vi "大富翁.vi"() -> ()   [LabVIEW 2014] (continued)
                                n1877 = stacked-sequence {
                                tunnel: [_ w1316] -> w1303
                                frame #0 {
                                n1878 = call "機會-500.vi"() -> ()  [unwired: 4 in]
                                n1879 = local read "換誰?"() -> (w1304:dbl)
                                n1880 = case shown="1, Default" w1304 {
                                tunnel: [w1312 w1313 w1314 w1315] -> w1305
                                frame 1, Default {
                                n1881 = local read "玩家一財產"() -> (w1312:dbl)
                                }
                                frame 2 {
                                n1882 = local read "玩家二財產"() -> (w1313:dbl)
                                }
                                frame 3 {
                                n1883 = local read "玩家三財產"() -> (w1314:dbl)
                                }
                                frame 4 {
                                n1884 = local read "玩家四財產"() -> (w1315:dbl)
                                }
                                }
                                n1885 = Subtract(x=w1305, y=500.0) -> (x-y=w1307:dbl)
                                n1886 = case shown="1, Default" w1304 {
                                tunnel: w1307 -> [w1308 w1309 w1310 w1311]
                                frame 1, Default {
                                n1887 = local write "玩家一財產"(w1308) -> ()
                                }
                                frame 2 {
                                n1888 = local write "玩家二財產"(w1309) -> ()
                                }
                                frame 3 {
                                n1889 = local write "玩家三財產"(w1310) -> ()
                                }
                                frame 4 {
                                n1890 = local write "玩家四財產"(w1311) -> ()
                                }
                                }
                                }
                                frame #1 {
                                n1891 = local read "換誰?"() -> (w1318:dbl)
                                n1892 = case shown="1, Default" w1318 {
                                tunnel: [w1322 w1323 w1324 w1325] -> w1319
                                frame 1, Default {
                                n1893 = local read "玩家一財產"() -> (w1322:dbl)
                                }
                                frame 2 {
                                n1894 = local read "玩家二財產"() -> (w1323:dbl)
                                }
                                frame 3 {
                                n1895 = local read "玩家三財產"() -> (w1324:dbl)
                                }
                                frame 4 {
                                n1896 = local read "玩家四財產"() -> (w1325:dbl)
                                }
                                }
                                n1897 = Less Than 0?(x=w1319) -> (x < 0?=w1317:bool)
                                n1898 = case shown="True" w1317 {
                                tunnel: [FALSE TRUE] -> w1316
                                frame False {
                                }
                                frame True {
                                n1899 = call "破產了.vi"() -> ()  [unwired: 4 in]
                                }
                                }
                                }
                                }
                                }
                                }
                                }
                                frame True {
                                # "58~60"
                                n1900 = call "機會全部+3000.vi"() -> ()  [unwired: 4 in]
                                n1901 = local read "玩家三財產"() -> (w1330:dbl)
                                n1902 = local read "玩家二財產"() -> (w1332:dbl)
                                n1903 = local read "玩家一財產"() -> (w1334:dbl)
                                n1904 = Add(x=w1330, y=3000.0) -> (x+y=w1329:dbl)
                                n1905 = Add(x=w1332, y=3000.0) -> (x+y=w1331:dbl)
                                n1906 = local read "玩家四財產"() -> (w1328:dbl)
                                n1907 = Add(x=w1334, y=3000.0) -> (x+y=w1333:dbl)
                                n1908 = Add(x=w1328, y=3000.0) -> (x+y=w1327:dbl)
                                n1909 = local write "玩家三財產"(w1329) -> ()
                                n1910 = local write "玩家二財產"(w1331) -> ()
                                n1911 = local write "玩家四財產"(w1327) -> ()
                                n1912 = local write "玩家一財產"(w1333) -> ()
                                }
                                }
                                }
                                frame True {
                                # "54~58"
                                n1913 = call "機會+3000.vi"() -> ()  [unwired: 4 in]
                                n1914 = local read "換誰?"() -> (w1340:dbl)
                                n1915 = case shown="1, Default" w1340 {
                                tunnel: [w1348 w1349 w1350 w1351] -> w1341
                                frame 1, Default {
                                n1916 = local read "玩家一財產"() -> (w1348:dbl)
                                }
                                frame 2 {
                                n1917 = local read "玩家二財產"() -> (w1349:dbl)
                                }
                                frame 3 {
                                n1918 = local read "玩家三財產"() -> (w1350:dbl)
                                }
                                frame 4 {
                                n1919 = local read "玩家四財產"() -> (w1351:dbl)
                                }
                                }
                                n1920 = Add(x=w1341, y=3000.0) -> (x+y=w1343:dbl)
                                n1921 = case shown="1, Default" w1340 {
                                tunnel: w1343 -> [w1344 w1345 w1346 w1347]
                                frame 1, Default {
                                n1922 = local write "玩家一財產"(w1344) -> ()
                                }
                                frame 2 {
                                n1923 = local write "玩家二財產"(w1345) -> ()
                                }
                                frame 3 {
                                n1924 = local write "玩家三財產"(w1346) -> ()
                                }
                                frame 4 {
                                n1925 = local write "玩家四財產"(w1347) -> ()
                                }
                                }
                                }
                                }
                                }
                                frame True {
                                # "45~54"
                                n1926 = call "機會+2000.vi"() -> ()  [unwired: 4 in]
                                n1927 = local read "換誰?"() -> (w1353:dbl)
                                n1928 = case shown="1, Default" w1353 {
                                tunnel: [w1361 w1362 w1363 w1364] -> w1354
                                frame 1, Default {
                                n1929 = local read "玩家一財產"() -> (w1361:dbl)
                                }
                                frame 2 {
                                n1930 = local read "玩家二財產"() -> (w1362:dbl)
                                }
                                frame 3 {
                                n1931 = local read "玩家三財產"() -> (w1363:dbl)
                                }
                                frame 4 {
                                n1932 = local read "玩家四財產"() -> (w1364:dbl)
                                }
                                }
                                n1933 = Add(x=w1354, y=2000.0) -> (x+y=w1356:dbl)
                                n1934 = case shown="1, Default" w1353 {
                                tunnel: w1356 -> [w1357 w1358 w1359 w1360]
                                frame 1, Default {
                                n1935 = local write "玩家一財產"(w1357) -> ()
                                }
                                frame 2 {
                                n1936 = local write "玩家二財產"(w1358) -> ()
                                }
                                frame 3 {
                                n1937 = local write "玩家三財產"(w1359) -> ()
                                }
                                frame 4 {
                                n1938 = local write "玩家四財產"(w1360) -> ()
                                }
                                }
                                }
                                }
                                }
                                frame True {
                                # "30~45"
                                n1939 = call "機會+1000.vi"() -> ()  [unwired: 4 in]
                                n1940 = local read "換誰?"() -> (w1366:dbl)
                                n1941 = case shown="1, Default" w1366 {
                                tunnel: [w1374 w1375 w1376 w1377] -> w1367
                                frame 1, Default {
                                n1942 = local read "玩家一財產"() -> (w1374:dbl)
                                }
                                frame 2 {
                                n1943 = local read "玩家二財產"() -> (w1375:dbl)
                                }
                                frame 3 {
                                n1944 = local read "玩家三財產"() -> (w1376:dbl)
                                }
                                frame 4 {
                                n1945 = local read "玩家四財產"() -> (w1377:dbl)
                                }
                                }
                                n1946 = Add(x=w1367, y=1000.0) -> (x+y=w1369:dbl)
                                n1947 = case shown="1, Default" w1366 {
                                tunnel: w1369 -> [w1370 w1371 w1372 w1373]
                                frame 1, Default {
                                n1948 = local write "玩家一財產"(w1370) -> ()
                                }
                                frame 2 {
                                n1949 = local write "玩家二財產"(w1371) -> ()
                                }
                                frame 3 {
                                n1950 = local write "玩家三財產"(w1372) -> ()
                                }
                                frame 4 {
                                n1951 = local write "玩家四財產"(w1373) -> ()
                                }
                                }
                                }
                                }
                              }
                              frame True {
                                # "10~30"
                                n1952 = call "機會+500.vi"() -> ()  [unwired: 4 in]
                                n1953 = local read "換誰?"() -> (w1382:dbl)
                                n1954 = case shown="1, Default" w1382 {
                                tunnel: [w1387 w1388 w1389 w1390] -> w1381
                                frame 1, Default {
                                n1955 = local read "玩家一財產"() -> (w1387:dbl)
                                }
                                frame 2 {
                                n1956 = local read "玩家二財產"() -> (w1388:dbl)
                                }
                                frame 3 {
                                n1957 = local read "玩家三財產"() -> (w1389:dbl)
                                }
                                frame 4 {
                                n1958 = local read "玩家四財產"() -> (w1390:dbl)
                                }
                                }
                                n1959 = Add(x=w1381, y=500.0) -> (x+y=w1379:dbl)
                                n1960 = case shown="4" w1382 {
                                tunnel: w1379 -> [w1383 w1384 w1385 w1386]
                                frame 1, Default {
                                n1961 = local write "玩家一財產"(w1383) -> ()
                                }
                                frame 2 {
                                n1962 = local write "玩家二財產"(w1384) -> ()
                                }
                                frame 3 {
                                n1963 = local write "玩家三財產"(w1385) -> ()
                                }
                                frame 4 {
                                n1964 = local write "玩家四財產"(w1386) -> ()
                                }
                                }
                              }
                            }
                          }
                          frame True {
                            # "5~10%"
                            n1965 = local read "換誰?"() -> (w1392:dbl)
                            n1966 = case shown="1" w1392 {
                              frame 0, Default {
                              }
                              frame 1 {
                                n1967 = local write "剩幾天 1"(2.0 ("剩幾天 1")) -> ()
                                n1968 = local write "位置 1"(13.0 ("位置 1")) -> ()
                                n1969 = property on="入獄 1" class="Bool (strict)"("Visible"=TRUE) -> ()  [unwired: 2 in, 2 out]
                                n1970 = property on="P1 棋子" class="Bool (strict)"("Left"=1503 ("Position:Left"), "Top"=112 ("Position:Top")) -> ()  [unwired: 2 in, 2 out]
                              }
                              frame 2 {
                                n1971 = local write "位置 2"(13.0 ("位置 2")) -> ()
                                n1972 = local write "剩幾天 2"(2.0 ("剩幾天 2")) -> ()
                                n1973 = property on="入獄 2" class="Bool (strict)"("Visible"=TRUE) -> ()  [unwired: 2 in, 2 out]
                                n1974 = property on="P2 棋子" class="Bool (strict)"("Left"=1540 ("Position:Left"), "Top"=112 ("Position:Top")) -> ()  [unwired: 2 in, 2 out]
                              }
                              frame 3 {
                                n1975 = local write "剩幾天 3"(2.0 ("剩幾天 3")) -> ()
                                n1976 = local write "位置 3"(13.0 ("位置 3")) -> ()
                                n1977 = property on="入獄 3" class="Bool (strict)"("Visible"=TRUE) -> ()  [unwired: 2 in, 2 out]
                                n1978 = property on="P3 棋子" class="Bool (strict)"("Left"=1503 ("Position:Left"), "Top"=144 ("Position:Top")) -> ()  [unwired: 2 in, 2 out]
                              }
                              frame 4 {
                                n1979 = local write "剩幾天 4"(2.0 ("剩幾天 4")) -> ()
                                n1980 = local write "位置 4"(13.0 ("位置 4")) -> ()
                                n1981 = property on="入獄 4" class="Bool (strict)"("Visible"=TRUE) -> ()  [unwired: 2 in, 2 out]
                                n1982 = property on="P4 棋子" class="Bool (strict)"("Left"=1540 ("Position:Left"), "Top"=144 ("Position:Top")) -> ()  [unwired: 2 in, 2 out]
                              }
                            }
                            n1983 = call "32入獄.vi"() -> ()  [unwired: 4 in]
                          }
                        }
                      }
                      frame True {
                        # "2~5"
                        n1984 = local read "換誰?"() -> (w1414:dbl)
                        n1985 = case shown="1" w1414 {
                          frame 0, Default {
                          }
                          frame 1 {
                            n1986 = local write "剩幾天 1"(3.0 ("剩幾天 1")) -> ()
                            n1987 = local write "位置 1"(13.0 ("位置 1")) -> ()
                            n1988 = property on="入獄 1" class="Bool (strict)"("Visible"=TRUE) -> ()  [unwired: 2 in, 2 out]
                            n1989 = property on="P1 棋子" class="Bool (strict)"("Left"=1503 ("Position:Left"), "Top"=112 ("Position:Top")) -> ()  [unwired: 2 in, 2 out]
                          }
                          frame 2 {
                            n1990 = local write "位置 2"(13.0 ("位置 2")) -> ()
                            n1991 = local write "剩幾天 2"(3.0 ("剩幾天 2")) -> ()
                            n1992 = property on="入獄 2" class="Bool (strict)"("Visible"=TRUE) -> ()  [unwired: 2 in, 2 out]
                            n1993 = property on="P2 棋子" class="Bool (strict)"("Left"=1540 ("Position:Left"), "Top"=112 ("Position:Top")) -> ()  [unwired: 2 in, 2 out]
                          }
                          frame 3 {
                            n1994 = local write "剩幾天 3"(3.0 ("剩幾天 3")) -> ()
                            n1995 = local write "位置 3"(13.0 ("位置 3")) -> ()
                            n1996 = property on="入獄 3" class="Bool (strict)"("Visible"=TRUE) -> ()  [unwired: 2 in, 2 out]
                            n1997 = property on="P3 棋子" class="Bool (strict)"("Left"=1503 ("Position:Left"), "Top"=144 ("Position:Top")) -> ()  [unwired: 2 in, 2 out]
                          }
                          frame 4 {
                            n1998 = local write "剩幾天 4"(3.0 ("剩幾天 4")) -> ()
                            n1999 = local write "位置 4"(13.0 ("位置 4")) -> ()
                            n2000 = property on="入獄 4" class="Bool (strict)"("Visible"=TRUE) -> ()  [unwired: 2 in, 2 out]
                            n2001 = property on="P4 棋子" class="Bool (strict)"("Left"=1540 ("Position:Left"), "Top"=144 ("Position:Top")) -> ()  [unwired: 2 in, 2 out]
                          }
                        }
                        n2002 = call "入獄3天.vi"() -> ()  [unwired: 4 in]
                      }
                    }
                  }
                  frame True {
                    # "0~2%"
                    n2003 = stacked-sequence {
                      tunnel: [_ w1468] -> w1435
                      frame #0 {
                        n2004 = local read "換誰?"() -> (w1436:dbl)
                        n2005 = case shown="4" w1436 {
                          frame 0, Default {
                          }
                          frame 1 {
                            n2006 = local write "剩幾天 1"(5.0 ("剩幾天 1")) -> ()
                            n2007 = local write "位置 1"(13.0 ("位置 1")) -> ()
                            n2008 = property on="入獄 1" class="Bool (strict)"("Visible"=TRUE) -> ()  [unwired: 2 in, 2 out]
                            n2009 = property on="P1 棋子" class="Bool (strict)"("Left"=1503 ("Position:Left"), "Top"=112 ("Position:Top")) -> ()  [unwired: 2 in, 2 out]
                          }
                          frame 2 {
                            n2010 = local write "位置 2"(13.0 ("位置 2")) -> ()
                            n2011 = local write "剩幾天 2"(5.0 ("剩幾天 2")) -> ()
                            n2012 = property on="入獄 2" class="Bool (strict)"("Visible"=TRUE) -> ()  [unwired: 2 in, 2 out]
                            n2013 = property on="P2 棋子" class="Bool (strict)"("Left"=1540 ("Position:Left"), "Top"=112 ("Position:Top")) -> ()  [unwired: 2 in, 2 out]
                          }
                          frame 3 {
                            n2014 = local write "剩幾天 3"(5.0 ("剩幾天 3")) -> ()
                            n2015 = local write "位置 3"(13.0 ("位置 3")) -> ()
                            n2016 = property on="入獄 3" class="Bool (strict)"("Visible"=TRUE) -> ()  [unwired: 2 in, 2 out]
                            n2017 = property on="P3 棋子" class="Bool (strict)"("Left"=1503 ("Position:Left"), "Top"=144 ("Position:Top")) -> ()  [unwired: 2 in, 2 out]
                          }
                          frame 4 {
                            n2018 = local write "剩幾天 4"(5.0 ("剩幾天 4")) -> ()
                            n2019 = local write "位置 4"(13.0 ("位置 4")) -> ()
                            n2020 = property on="入獄 4" class="Bool (strict)"("Visible"=TRUE) -> ()  [unwired: 2 in, 2 out]
                            n2021 = property on="P4 棋子" class="Bool (strict)"("Left"=1540 ("Position:Left"), "Top"=144 ("Position:Top")) -> ()  [unwired: 2 in, 2 out]
                          }
                        }
                        n2022 = case shown="1, Default" w1436 {
                          tunnel: [w1444 w1445 w1446 w1447] -> w1439
                          frame 1, Default {
                            n2023 = local read "玩家一財產"() -> (w1444:dbl)
                          }
                          frame 2 {
                            n2024 = local read "玩家二財產"() -> (w1445:dbl)
                          }
                          frame 3 {
                            n2025 = local read "玩家三財產"() -> (w1446:dbl)
                          }
                          frame 4 {
                            n2026 = local read "玩家四財產"() -> (w1447:dbl)
                          }
                        }
                        n2027 = Subtract(x=w1439, y=2000.0) -> (x-y=w1437:dbl)
                        n2028 = case shown="4" w1436 {
                          tunnel: w1437 -> [w1440 w1441 w1442 w1443]
                          frame 1, Default {
                            n2029 = local write "玩家一財產"(w1440) -> ()
                          }
                          frame 2 {
                            n2030 = local write "玩家二財產"(w1441) -> ()
                          }
                          frame 3 {
                            n2031 = local write "玩家三財產"(w1442) -> ()
                          }
                          frame 4 {
                            n2032 = local write "玩家四財產"(w1443) -> ()
                          }
                        }
                        n2033 = call "入獄5天.vi"() -> ()  [unwired: 4 in]
                      }
                      frame #1 {
                        n2034 = local read "換誰?"() -> (w1470:dbl)
                        n2035 = case shown="1, Default" w1470 {
                          tunnel: [w1474 w1475 w1476 w1477] -> w1471
                          frame 1, Default {
                            n2036 = local read "玩家一財產"() -> (w1474:dbl)
                          }
                          frame 2 {
                            n2037 = local read "玩家二財產"() -> (w1475:dbl)
                          }
                          frame 3 {
                            n2038 = local read "玩家三財產"() -> (w1476:dbl)
                          }
                          frame 4 {
                            n2039 = local read "玩家四財產"() -> (w1477:dbl)
                          }
                        }
                        n2040 = Less Than 0?(x=w1471) -> (x < 0?=w1469:bool)
                        n2041 = case shown="True" w1469 {
                          tunnel: [FALSE TRUE] -> w1468
                          frame False {
                          }
                          frame True {
                            n2042 = call "破產了.vi"() -> ()  [unwired: 4 in]
                          }
                        }
                      }
                    }
                  }
                }
              }
              frame True {
                n2043 = local read "換誰?"() -> (w1479:dbl)
                n2044 = case shown="4" w1479 {
                  frame 0, Default {
                  }
                  frame 1 {
                    n2045 = local write "剩幾天 1"(2.0 ("剩幾天 1")) -> ()
                    n2046 = local write "位置 1"(13.0 ("位置 1")) -> ()
                    n2047 = property on="入獄 1" class="Bool (strict)"("Visible"=TRUE) -> ()  [unwired: 2 in, 2 out]
                    n2048 = property on="P1 棋子" class="Bool (strict)"("Left"=1503 ("Position:Left"), "Top"=112 ("Position:Top")) -> ()  [unwired: 2 in, 2 out]
                  }
                  frame 2 {
                    n2049 = local write "剩幾天 2"(2.0 ("剩幾天 2")) -> ()
                    n2050 = local write "位置 2"(13.0 ("位置 2")) -> ()
                    n2051 = property on="入獄 2" class="Bool (strict)"("Visible"=TRUE) -> ()  [unwired: 2 in, 2 out]
                    n2052 = property on="P2 棋子" class="Bool (strict)"("Left"=1540 ("Position:Left"), "Top"=112 ("Position:Top")) -> ()  [unwired: 2 in, 2 out]
                  }
                  frame 3 {
                    n2053 = local write "剩幾天 3"(2.0 ("剩幾天 3")) -> ()
                    n2054 = local write "位置 3"(13.0 ("位置 3")) -> ()
                    n2055 = local write "位置 3"(13.0 ("位置 3")) -> ()
                    n2056 = property on="入獄 3" class="Bool (strict)"("Visible"=TRUE) -> ()  [unwired: 2 in, 2 out]
                    n2057 = property on="P3 棋子" class="Bool (strict)"("Left"=1503 ("Position:Left"), "Top"=144 ("Position:Top")) -> ()  [unwired: 2 in, 2 out]
                  }
                  frame 4 {
                    n2058 = local write "位置 4"(13.0 ("位置 4")) -> ()
                    n2059 = local write "剩幾天 4"(2.0 ("剩幾天 4")) -> ()
                    n2060 = property on="入獄 4" class="Bool (strict)"("Visible"=TRUE) -> ()  [unwired: 2 in, 2 out]
                    n2061 = property on="P4 棋子" class="Bool (strict)"("Left"=1540 ("Position:Left"), "Top"=144 ("Position:Top")) -> ()  [unwired: 2 in, 2 out]
                  }
                }
                n2062 = call "32入獄.vi"() -> ()  [unwired: 4 in]
              }
            }
          }
          frame 9 {
            n2063 = local read "台東縣所有"() -> (w1501:u32)
            n2064 = Equal?(x=w1501, y=u32 16777215) -> (x = y?=w1504:bool)
            n2065 = case shown="False" w1504 {
              tunnel: w1503 -> [w1528 w1565]
              tunnel: [w1518 FALSE] -> w1502
              frame False {
                # "有主地"
                n2066 = local read "換誰?"() -> (w1521:dbl)
                n2067 = local read "台東縣所有"() -> (w1507:u32)
                n2068 = call "數字轉顏色.vi"("數字"=w1521) -> ("顏色數字"=w1508:dbl)  [unwired: 2 in]
                n2069 = case shown="4" w1521 {
                  tunnel: [w1560 w1561 w1562 w1563] -> w1527
                  frame 1, Default {
                    n2070 = local read "玩家一財產"() -> (w1560:dbl)
                  }
                  frame 2 {
                    n2071 = local read "玩家二財產"() -> (w1561:dbl)
                  }
                  frame 3 {
                    n2072 = local read "玩家三財產"() -> (w1562:dbl)
                  }
                  frame 4 {
                    n2073 = local read "玩家四財產"() -> (w1563:dbl)
                  }
                }
                n2074 = Equal?(x=w1507, y=w1508) -> (x = y?=w1531:bool)
                n2075 = local read "台東縣所有"() -> (w1509:u32)
                n2076 = local read "9旅4"() -> (w1517:bool)
                n2077 = local read "9旅3"() -> (w1516:bool)
                n2078 = local read "9旅2"() -> (w1515:bool)
                n2079 = local read "9旅1"() -> (w1514:bool)
                n2080 = local read "9房4"() -> (w1513:bool)
                n2081 = local read "9房3"() -> (w1512:bool)
                n2082 = local read "9房2"() -> (w1511:bool)
                n2083 = local read "9房1"() -> (w1510:bool)
                n2084 = call "房子數量.vi"("房子 1"=w1510, "房子 2"=w1511, "房子 3"=w1512, "房子 4"=w1513, "旅館 1"=w1514, "旅館 2"=w1515, "旅館 3"=w1516, "旅館 4"=w1517) -> ("房子數"=w1530:dbl, "旅館數"=w1529:dbl)  [unwired: 18 in]
                n2085 = call "顏色轉數字.vi"("顏色數字"=w1509) -> ("數字"=w1519:dbl)  [unwired: 2 in]
                n2086 = case shown="1, Default" w1519 {
                  tunnel: [w1536 w1537 w1538 w1539] -> w1523
                  frame 1, Default {
                    n2087 = local read "玩家一財產"() -> (w1536:dbl)
                  }
                  frame 2 {
                    n2088 = local read "玩家二財產"() -> (w1537:dbl)
                  }
                  frame 3 {
                    n2089 = local read "玩家三財產"() -> (w1538:dbl)
                  }
                  frame 4 {
                    n2090 = local read "玩家四財產"() -> (w1539:dbl)
                  }
                }
                n2091 = call "走到地.vi"("房子數量"=w1530, "自己的地?"=w1531, "旅館數量"=w1529, "編號"=w1528, "走到人財產"=w1527) -> ("走到人-?"=w1526:dbl, "蓋第幾棟"=w1524:dbl, "地主+?"=w1522:dbl, "破產?"=w1518:bool)
                n2092 = Subtract(x=w1527, y=w1526) -> (x-y=w1525:dbl)
                n2093 = Add(x=w1522, y=w1523) -> (x+y=w1520:dbl)
                n2094 = case shown="1, Default" w1519 {
                  tunnel: w1520 -> [w1532 w1533 w1534 w1535]
                  frame 1, Default {
                    n2095 = local write "玩家一財產"(w1532) -> ()
                  }
                  frame 2 {
                    n2096 = local write "玩家二財產"(w1533) -> ()
                  }
                  frame 3 {
                    n2097 = local write "玩家三財產"(w1534) -> ()
                  }
                  frame 4 {
                    n2098 = local write "玩家四財產"(w1535) -> ()
                  }
                }
                n2099 = case shown="8" w1524 {
                  frame 0, Default {
                  }
                  frame 1 {
                    n2100 = flat-sequence {
                      frame #0 {
                        n2101 = local write "9房1"(TRUE ("1房1")) -> ()
                      }
                      frame #1 {
                        n2102 = property on="9房1" class="Bool (strict)"("Visible"=TRUE) -> ()  [unwired: 2 in, 2 out]
                      }
                    }
                  }
                  frame 2 {
                    n2103 = flat-sequence {
                      frame #0 {
                        n2104 = local write "9房2"(TRUE ("1房2")) -> ()
                      }
                      frame #1 {
                        n2105 = property on="9房2" class="Bool (strict)"("Visible"=TRUE ("1房2")) -> ()  [unwired: 2 in, 2 out]
                      }
                    }
                  }
                  frame 3 {
                    n2106 = flat-sequence {
                      frame #0 {
                        n2107 = local write "9房3"(TRUE) -> ()
                      }
                      frame #1 {
                        n2108 = property on="9房3" class="Bool (strict)"("Visible"=TRUE) -> ()  [unwired: 2 in, 2 out]
                      }
                    }
                  }
                  frame 4 {
                    n2109 = flat-sequence {
                      frame #0 {
                        n2110 = local write "9房4"(TRUE) -> ()
                      }
                      frame #1 {
                        n2111 = property on="9房4" class="Bool (strict)"("Visible"=TRUE) -> ()  [unwired: 2 in, 2 out]
                      }
                    }
                  }
                  frame 5 {
                    n2112 = flat-sequence {
                      frame #0 {
                        n2113 = local write "9旅1"(TRUE) -> ()
                      }
                      frame #1 {
                        n2114 = property on="9旅1" class="Bool (strict)"("Visible"=TRUE) -> ()  [unwired: 2 in, 2 out]
                      }
                    }
                  }
                  frame 6 {
                    n2115 = flat-sequence {
                      frame #0 {
                        n2116 = local write "9旅2"(TRUE) -> ()
                      }
                      frame #1 {
                        n2117 = property on="9旅2" class="Bool (strict)"("Visible"=TRUE) -> ()  [unwired: 2 in, 2 out]
                      }
                    }
                  }
                  frame 7 {
                    n2118 = flat-sequence {
                      frame #0 {
                        n2119 = local write "9旅3"(TRUE) -> ()
                      }
                      frame #1 {
                        n2120 = property on="9旅3" class="Bool (strict)"("Visible"=TRUE) -> ()  [unwired: 2 in, 2 out]
                      }
                    }
                  }
                  frame 8 {
                    n2121 = flat-sequence {
                      frame #0 {
                        n2122 = local write "9旅4"(TRUE) -> ()
                      }
                      frame #1 {
                        n2123 = property on="9旅4" class="Bool (strict)"("Visible"=TRUE) -> ()  [unwired: 2 in, 2 out]
                      }
                    }
                  }
                }
                n2124 = case shown="1, Default" w1521 {
                  tunnel: w1525 -> [w1556 w1557 w1558 w1559]
                  frame 1, Default {
                    n2125 = local write "玩家一財產"(w1556) -> ()
                  }
                  frame 2 {
                    n2126 = local write "玩家二財產"(w1557) -> ()
                  }
                  frame 3 {
                    n2127 = local write "玩家三財產"(w1558) -> ()
                  }
                  frame 4 {
                    n2128 = local write "玩家四財產"(w1559) -> ()
                  }
                }
              }
              frame True {
                # "無主地"
                n2129 = call "購買土地.vi"() -> ("確定 2"=w1566:bool)  [unwired: 3 in]
                n2130 = case shown="True" w1566 {
                  tunnel: w1565 -> [_ w1570]
                  frame False {
                    # "不買"
                  }
                  frame True {
                    # "要買"
                    n2131 = local read "換誰?"() -> (w1571:dbl)
                    n2132 = case shown="4" w1571 {
                      tunnel: [w1598 w1599 w1600 w1601] -> w1569
                      frame 1, Default {
                        n2133 = local read "玩家一財產"() -> (w1598:dbl)
                      }
                      frame 2 {
                        n2134 = local read "玩家二財產"() -> (w1599:dbl)
                      }
                      frame 3 {
                        n2135 = local read "玩家三財產"() -> (w1600:dbl)
                      }
                      frame 4 {
                        n2136 = local read "玩家四財產"() -> (w1601:dbl)
                      }
                    }
                    n2137 = call "各種價格.vi"("Numeric"=w1570) -> ("買空地"=w1568:dbl)  [unwired: 4 in, 5 out]
                    n2138 = Greater Or Equal?(x=w1569, y=w1568) -> (x >= y?=w1567:bool)
                    n2139 = case shown="True" w1567 {
                      tunnel: w1570 -> [_ w1572]
                      frame False {
                        # "錢不夠"
                        n2140 = call "錢不夠.vi"() -> ()  [unwired: 4 in]
                      }
                      frame True {
                        # "錢夠"
                        n2141 = local read "換誰?"() -> (w1573:dbl)
                        n2142 = case shown="3" w1573 {
                          selector: w1573 -> [w1577 w1583 w1589 w1595]
                          tunnel: w1572 -> [w1576 w1582 w1588 w1594]
                          frame 1, Default {
                            # "誰買了地"
                            n2143 = call "各種價格.vi"("Numeric"=w1576) -> ("買空地"=w1575:dbl)  [unwired: 4 in, 5 out]
                            n2144 = local read "玩家一財產"() -> (w1579:dbl)
                            n2145 = Subtract(x=w1579, y=w1575) -> (x-y=w1578:dbl)
                            n2146 = local write "玩家一財產"(w1578) -> ()
                            n2147 = call "數字轉顏色.vi"("數字"=w1577) -> ("顏色數字"=w1574:dbl)  [unwired: 2 in]
                            n2148 = local write "9台東縣"(w1574) -> ()
                            n2149 = local write "台東縣所有"(w1574) -> ()
                          }
                          frame 2 {
                            # "誰買了地"
                            n2150 = call "各種價格.vi"("Numeric"=w1582) -> ("買空地"=w1581:dbl)  [unwired: 4 in, 5 out]
                            n2151 = local read "玩家二財產"() -> (w1585:dbl)
                            n2152 = Subtract(x=w1585, y=w1581) -> (x-y=w1584:dbl)
                            n2153 = local write "玩家二財產"(w1584) -> ()
                            n2154 = call "數字轉顏色.vi"("數字"=w1583) -> ("顏色數字"=w1580:dbl)  [unwired: 2 in]
                            n2155 = local write "9台東縣"(w1580) -> ()
                            n2156 = local write "台東縣所有"(w1580) -> ()
                          }
                          frame 3 {
                            # "誰買了地"
                            n2157 = local read "玩家三財產"() -> (w1590:dbl)
                            n2158 = call "各種價格.vi"("Numeric"=w1588) -> ("買空地"=w1587:dbl)  [unwired: 4 in, 5 out]
                            n2159 = Subtract(x=w1590, y=w1587) -> (x-y=w1591:dbl)
                            n2160 = call "數字轉顏色.vi"("數字"=w1589) -> ("顏色數字"=w1586:dbl)  [unwired: 2 in]
                            n2161 = local write "玩家三財產"(w1591) -> ()
                            n2162 = local write "9台東縣"(w1586) -> ()
                            n2163 = local write "台東縣所有"(w1586) -> ()
                          }
                          frame 4 {
                            # "誰買了地"
                            n2164 = call "各種價格.vi"("Numeric"=w1594) -> ("買空地"=w1593:dbl)  [unwired: 4 in, 5 out]
                            n2165 = local read "玩家四財產"() -> (w1597:dbl)
                            n2166 = Subtract(x=w1597, y=w1593) -> (x-y=w1596:dbl)
                            n2167 = local write "玩家四財產"(w1596) -> ()
                            n2168 = call "數字轉顏色.vi"("數字"=w1595) -> ("顏色數字"=w1592:dbl)  [unwired: 2 in]
                            n2169 = local write "9台東縣"(w1592) -> ()
                            n2170 = local write "台東縣所有"(w1592) -> ()
                          }
                        }
                      }
                    }
                  }
                }
              }
            }
          }
          frame 10 {
            n2171 = local read "綠島所有"() -> (w1602:u32)
            n2172 = Equal?(x=w1602, y=u32 16777215) -> (x = y?=w1605:bool)
            n2173 = case shown="True" w1605 {
              tunnel: w1604 -> [w1628 w1666]
              tunnel: [w1618 FALSE] -> w1603
              frame False {
                # "有主地"
                n2174 = local read "換誰?"() -> (w1621:dbl)
                n2175 = local read "綠島所有"() -> (w1609:u32)
                n2176 = call "數字轉顏色.vi"("數字"=w1621) -> ("顏色數字"=w1632:dbl)  [unwired: 2 in]
                n2177 = case shown="4" w1621 {
                  tunnel: [w1661 w1662 w1663 w1664] -> w1627
                  frame 1, Default {
                    n2178 = local read "玩家一財產"() -> (w1661:dbl)
                  }
                  frame 2 {
                    n2179 = local read "玩家二財產"() -> (w1662:dbl)
                  }
                  frame 3 {
                    n2180 = local read "玩家三財產"() -> (w1663:dbl)
                  }
                  frame 4 {
                    n2181 = local read "玩家四財產"() -> (w1664:dbl)
                  }
                }
                n2182 = Equal?(x=w1609, y=w1632) -> (x = y?=w1631:bool)
                n2183 = local read "綠島所有"() -> (w1608:u32)
                n2184 = local read "10旅4"() -> (w1617:bool)
                n2185 = local read "10旅3"() -> (w1616:bool)
                n2186 = local read "10旅2"() -> (w1615:bool)
                n2187 = local read "10旅1"() -> (w1614:bool)
                n2188 = local read "10房4"() -> (w1613:bool)
                n2189 = local read "10房3"() -> (w1612:bool)
                n2190 = local read "10房2"() -> (w1611:bool)
                n2191 = local read "10房1"() -> (w1610:bool)
                n2192 = call "房子數量.vi"("房子 1"=w1610, "房子 2"=w1611, "房子 3"=w1612, "房子 4"=w1613, "旅館 1"=w1614, "旅館 2"=w1615, "旅館 3"=w1616, "旅館 4"=w1617) -> ("房子數"=w1630:dbl, "旅館數"=w1629:dbl)  [unwired: 18 in]
                n2193 = call "顏色轉數字.vi"("顏色數字"=w1608) -> ("數字"=w1619:dbl)  [unwired: 2 in]
                n2194 = case shown="1, Default" w1619 {
                  tunnel: [w1637 w1638 w1639 w1640] -> w1623
                  frame 1, Default {
                    n2195 = local read "玩家一財產"() -> (w1637:dbl)
                  }
                  frame 2 {
                    n2196 = local read "玩家二財產"() -> (w1638:dbl)
                  }
                  frame 3 {
                    n2197 = local read "玩家三財產"() -> (w1639:dbl)
                  }
                  frame 4 {
                    n2198 = local read "玩家四財產"() -> (w1640:dbl)
                  }
                }
                n2199 = call "走到地.vi"("房子數量"=w1630, "自己的地?"=w1631, "旅館數量"=w1629, "編號"=w1628, "走到人財產"=w1627) -> ("走到人-?"=w1626:dbl, "蓋第幾棟"=w1624:dbl, "地主+?"=w1622:dbl, "破產?"=w1618:bool)
                n2200 = Subtract(x=w1627, y=w1626) -> (x-y=w1625:dbl)
                n2201 = Add(x=w1622, y=w1623) -> (x+y=w1620:dbl)
                n2202 = case shown="1, Default" w1619 {
                  tunnel: w1620 -> [w1633 w1634 w1635 w1636]
                  frame 1, Default {
                    n2203 = local write "玩家一財產"(w1633) -> ()
                  }
                  frame 2 {
                    n2204 = local write "玩家二財產"(w1634) -> ()
                  }
                  frame 3 {
                    n2205 = local write "玩家三財產"(w1635) -> ()
                  }
                  frame 4 {
                    n2206 = local write "玩家四財產"(w1636) -> ()
                  }
                }
                n2207 = case shown="8" w1624 {
                  frame 0, Default {
                  }
                  frame 1 {
                    n2208 = flat-sequence {
                      frame #0 {
                        n2209 = local write "10房1"(TRUE ("1房1")) -> ()
                      }
                      frame #1 {
                        n2210 = property on="10房1" class="Bool (strict)"("Visible"=TRUE) -> ()  [unwired: 2 in, 2 out]
                      }
                    }
                  }
                  frame 2 {
                    n2211 = flat-sequence {
                      frame #0 {
                        n2212 = local write "10房2"(TRUE ("1房2")) -> ()
                      }
                      frame #1 {
                        n2213 = property on="10房2" class="Bool (strict)"("Visible"=TRUE ("1房2")) -> ()  [unwired: 2 in, 2 out]
                      }
                    }
                  }
                  frame 3 {
                    n2214 = flat-sequence {
                      frame #0 {
                        n2215 = local write "10房3"(TRUE) -> ()
                      }
                      frame #1 {
                        n2216 = property on="10房3" class="Bool (strict)"("Visible"=TRUE) -> ()  [unwired: 2 in, 2 out]
                      }
                    }
                  }
                  frame 4 {
                    n2217 = flat-sequence {
                      frame #0 {
                        n2218 = local write "10房4"(TRUE) -> ()
                      }
                      frame #1 {
                        n2219 = property on="10房4" class="Bool (strict)"("Visible"=TRUE) -> ()  [unwired: 2 in, 2 out]
                      }
                    }
                  }
                  frame 5 {
                    n2220 = flat-sequence {
                      frame #0 {
                        n2221 = local write "10旅1"(TRUE) -> ()
                      }
                      frame #1 {
                        n2222 = property on="10旅1" class="Bool (strict)"("Visible"=TRUE) -> ()  [unwired: 2 in, 2 out]
                      }
                    }
                  }
                  frame 6 {
                    n2223 = flat-sequence {
                      frame #0 {
                        n2224 = local write "10旅2"(TRUE) -> ()
                      }
                      frame #1 {
                        n2225 = property on="10旅2" class="Bool (strict)"("Visible"=TRUE) -> ()  [unwired: 2 in, 2 out]
                      }
                    }
                  }
                  frame 7 {
                    n2226 = flat-sequence {
                      frame #0 {
                        n2227 = local write "10旅3"(TRUE) -> ()
                      }
                      frame #1 {
                        n2228 = property on="10旅3" class="Bool (strict)"("Visible"=TRUE) -> ()  [unwired: 2 in, 2 out]
                      }
                    }
                  }
                  frame 8 {
                    n2229 = flat-sequence {
                      frame #0 {
                        n2230 = local write "10旅4"(TRUE) -> ()
                      }
                      frame #1 {
                        n2231 = property on="10旅4" class="Bool (strict)"("Visible"=TRUE) -> ()  [unwired: 2 in, 2 out]
                      }
                    }
                  }
                }
                n2232 = case shown="1, Default" w1621 {
                  tunnel: w1625 -> [w1657 w1658 w1659 w1660]
                  frame 1, Default {
                    n2233 = local write "玩家一財產"(w1657) -> ()
                  }
                  frame 2 {
                    n2234 = local write "玩家二財產"(w1658) -> ()
                  }
                  frame 3 {
                    n2235 = local write "玩家三財產"(w1659) -> ()
                  }
                  frame 4 {
                    n2236 = local write "玩家四財產"(w1660) -> ()
                  }
                }
              }
              frame True {
                # "無主地"
                n2237 = call "購買土地.vi"() -> ("確定 2"=w1667:bool)  [unwired: 3 in]
                n2238 = case shown="True" w1667 {
                  tunnel: w1666 -> [_ w1671]
                  frame False {
                    # "不買"
                  }
                  frame True {
                    # "要買"
                    n2239 = local read "換誰?"() -> (w1672:dbl)
                    n2240 = case shown="4" w1672 {
                      tunnel: [w1699 w1700 w1701 w1702] -> w1670
                      frame 1, Default {
                        n2241 = local read "玩家一財產"() -> (w1699:dbl)
                      }
                      frame 2 {
                        n2242 = local read "玩家二財產"() -> (w1700:dbl)
                      }
                      frame 3 {
                        n2243 = local read "玩家三財產"() -> (w1701:dbl)
                      }
                      frame 4 {
                        n2244 = local read "玩家四財產"() -> (w1702:dbl)
                      }
                    }
                    n2245 = call "各種價格.vi"("Numeric"=w1671) -> ("買空地"=w1669:dbl)  [unwired: 4 in, 5 out]
                    n2246 = Greater Or Equal?(x=w1670, y=w1669) -> (x >= y?=w1668:bool)
                    n2247 = case shown="True" w1668 {
                      tunnel: w1671 -> [_ w1673]
                      frame False {
                        # "錢不夠"
                        n2248 = call "錢不夠.vi"() -> ()  [unwired: 4 in]
                      }
                      frame True {
                        # "錢夠"
                        n2249 = local read "換誰?"() -> (w1674:dbl)
                        n2250 = case shown="3" w1674 {
                          selector: w1674 -> [w1678 w1684 w1690 w1696]
                          tunnel: w1673 -> [w1677 w1683 w1689 w1695]
                          frame 1, Default {
                            # "誰買了地"
                            n2251 = call "各種價格.vi"("Numeric"=w1677) -> ("買空地"=w1676:dbl)  [unwired: 4 in, 5 out]
                            n2252 = local read "玩家一財產"() -> (w1680:dbl)
                            n2253 = Subtract(x=w1680, y=w1676) -> (x-y=w1679:dbl)
                            n2254 = local write "玩家一財產"(w1679) -> ()
                            n2255 = call "數字轉顏色.vi"("數字"=w1678) -> ("顏色數字"=w1675:dbl)  [unwired: 2 in]
                            n2256 = local write "10綠島"(w1675) -> ()
                            n2257 = local write "綠島所有"(w1675) -> ()
                          }
                          frame 2 {
                            # "誰買了地"
                            n2258 = call "各種價格.vi"("Numeric"=w1683) -> ("買空地"=w1682:dbl)  [unwired: 4 in, 5 out]
                            n2259 = local read "玩家二財產"() -> (w1686:dbl)
                            n2260 = Subtract(x=w1686, y=w1682) -> (x-y=w1685:dbl)
                            n2261 = local write "玩家二財產"(w1685) -> ()
                            n2262 = call "數字轉顏色.vi"("數字"=w1684) -> ("顏色數字"=w1681:dbl)  [unwired: 2 in]
                            n2263 = local write "10綠島"(w1681) -> ()
                            n2264 = local write "綠島所有"(w1681) -> ()
                          }
                          frame 3 {
                            # "誰買了地"
                            n2265 = local read "玩家三財產"() -> (w1691:dbl)
                            n2266 = call "各種價格.vi"("Numeric"=w1689) -> ("買空地"=w1688:dbl)  [unwired: 4 in, 5 out]
                            n2267 = Subtract(x=w1691, y=w1688) -> (x-y=w1692:dbl)
                            n2268 = call "數字轉顏色.vi"("數字"=w1690) -> ("顏色數字"=w1687:dbl)  [unwired: 2 in]
                            n2269 = local write "玩家三財產"(w1692) -> ()
                            n2270 = local write "10綠島"(w1687) -> ()
                            n2271 = local write "綠島所有"(w1687) -> ()
                          }
                          frame 4 {
                            # "誰買了地"
                            n2272 = call "各種價格.vi"("Numeric"=w1695) -> ("買空地"=w1694:dbl)  [unwired: 4 in, 5 out]
                            n2273 = local read "玩家四財產"() -> (w1698:dbl)
                            n2274 = Subtract(x=w1698, y=w1694) -> (x-y=w1697:dbl)
                            n2275 = local write "玩家四財產"(w1697) -> ()
                            n2276 = call "數字轉顏色.vi"("數字"=w1696) -> ("顏色數字"=w1693:dbl)  [unwired: 2 in]
                            n2277 = local write "10綠島"(w1693) -> ()
                            n2278 = local write "綠島所有"(w1693) -> ()
                          }
                        }
                      }
                    }
                  }
                }
              }
            }
          }
          frame 11 {
            n2279 = local read "蘭嶼所有"() -> (w1703:u32)
            n2280 = Equal?(x=w1703, y=u32 16777215) -> (x = y?=w1706:bool)
            n2281 = case shown="False" w1706 {
              tunnel: w1705 -> [w1729 w1767]
              tunnel: [w1719 FALSE] -> w1704
              frame False {
                # "有主地"
                n2282 = local read "換誰?"() -> (w1722:dbl)
                n2283 = local read "蘭嶼所有"() -> (w1709:u32)
                n2284 = call "數字轉顏色.vi"("數字"=w1722) -> ("顏色數字"=w1733:dbl)  [unwired: 2 in]
                n2285 = case shown="4" w1722 {
                  tunnel: [w1762 w1763 w1764 w1765] -> w1728
                  frame 1, Default {
                    n2286 = local read "玩家一財產"() -> (w1762:dbl)
                  }
                  frame 2 {
                    n2287 = local read "玩家二財產"() -> (w1763:dbl)
                  }
                  frame 3 {
                    n2288 = local read "玩家三財產"() -> (w1764:dbl)
                  }
                  frame 4 {
                    n2289 = local read "玩家四財產"() -> (w1765:dbl)
                  }
                }
                n2290 = Equal?(x=w1709, y=w1733) -> (x = y?=w1732:bool)
                n2291 = local read "蘭嶼所有"() -> (w1710:u32)
                n2292 = local read "11旅4"() -> (w1711:bool)
                n2293 = local read "11旅3"() -> (w1712:bool)
                n2294 = local read "11旅2"() -> (w1713:bool)
                n2295 = local read "11旅1"() -> (w1714:bool)
                n2296 = local read "11房4"() -> (w1715:bool)
                n2297 = local read "11房3"() -> (w1716:bool)
                n2298 = local read "11房2"() -> (w1717:bool)
                n2299 = local read "11房1"() -> (w1718:bool)
                n2300 = call "房子數量.vi"("房子 1"=w1718, "房子 2"=w1717, "房子 3"=w1716, "房子 4"=w1715, "旅館 1"=w1714, "旅館 2"=w1713, "旅館 3"=w1712, "旅館 4"=w1711) -> ("房子數"=w1731:dbl, "旅館數"=w1730:dbl)  [unwired: 18 in]
                n2301 = call "顏色轉數字.vi"("顏色數字"=w1710) -> ("數字"=w1720:dbl)  [unwired: 2 in]
                n2302 = case shown="1, Default" w1720 {
                  tunnel: [w1738 w1739 w1740 w1741] -> w1724
                  frame 1, Default {
                    n2303 = local read "玩家一財產"() -> (w1738:dbl)
                  }
                  frame 2 {
                    n2304 = local read "玩家二財產"() -> (w1739:dbl)
                  }
                  frame 3 {
                    n2305 = local read "玩家三財產"() -> (w1740:dbl)
                  }
                  frame 4 {
                    n2306 = local read "玩家四財產"() -> (w1741:dbl)
                  }
                }
                n2307 = call "走到地.vi"("房子數量"=w1731, "自己的地?"=w1732, "旅館數量"=w1730, "編號"=w1729, "走到人財產"=w1728) -> ("走到人-?"=w1727:dbl, "蓋第幾棟"=w1725:dbl, "地主+?"=w1723:dbl, "破產?"=w1719:bool)
                n2308 = Subtract(x=w1728, y=w1727) -> (x-y=w1726:dbl)
                n2309 = Add(x=w1723, y=w1724) -> (x+y=w1721:dbl)
                n2310 = case shown="1, Default" w1720 {
                  tunnel: w1721 -> [w1734 w1735 w1736 w1737]
                  frame 1, Default {
                    n2311 = local write "玩家一財產"(w1734) -> ()
                  }
                  frame 2 {
                    n2312 = local write "玩家二財產"(w1735) -> ()
                  }
                  frame 3 {
                    n2313 = local write "玩家三財產"(w1736) -> ()
                  }
                  frame 4 {
                    n2314 = local write "玩家四財產"(w1737) -> ()
                  }
                }
                n2315 = case shown="8" w1725 {
                  frame 0, Default {
                  }
                  frame 1 {
                    n2316 = flat-sequence {
                      frame #0 {
                        n2317 = local write "11房1"(TRUE ("1房1")) -> ()
                      }
                      frame #1 {
